vi "CtrlAll.vi"(11 "SRE Enum":enum16{"Start", "Run", "End"}(ring)) -> ()   [LabVIEW 2014]
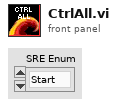
[diagram p1: front panel]
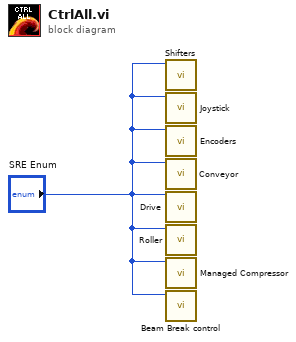
[diagram p0: block diagram]
diagram:
  n1 = call "Shifters.vi"("Enum"="SRE Enum") -> ()  [unwired: 11 in]
  n2 = call "Joystick.vi"("Enum"="SRE Enum") -> ()  [unwired: 9 in, 2 out]
  n3 = call "Encoders.vi"("Enum"="SRE Enum") -> ()  [unwired: 5 in, 6 out]
  n4 = call "Conveyor.vi"("Enum"="SRE Enum") -> ()  [unwired: 11 in]
  n5 = call "Drive.vi"("Enum"="SRE Enum") -> ()  [unwired: 15 in]
  n6 = call "Roller.vi"("Enum"="SRE Enum") -> ()  [unwired: 11 in]
  n7 = call "Managed Compressor.vi"("Enum"="SRE Enum") -> ()  [unwired: 11 in]
  n8 = call "Beam Break control.vi"("SRE ENUM"="SRE Enum") -> ()  [unwired: 9 in, 2 out]
